vi "Example Feedbacknode 1.vi"() -> ()   [LabVIEW 2014]
panel:
  out "Error Out":errorcluster
  in  "Error In":errorcluster
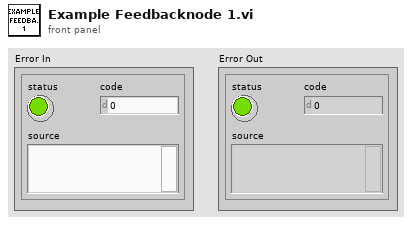
[diagram p1: front panel]
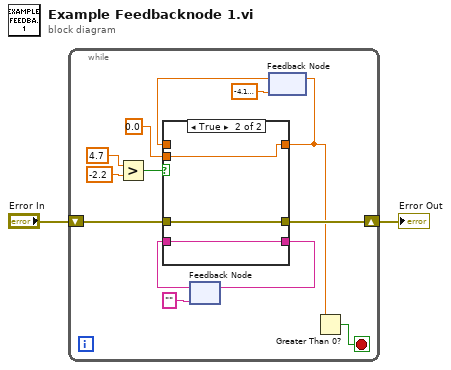
[diagram p0: block diagram]
diagram:
  n1 = while {
    shift-right: [w15] -> w2
    shift-left: "Error In" -> [w14]
    stop <- w4 stop-if-true
    n2 = Greater?(x=4.7, y=-2.2) -> (0:w13:bool)
    n3 = feedback #1("") -> (w6:string)
    n4 = feedback #2(sgl -4.2) -> (w8:sgl)
    n5 = case shown="True" w13 {
      tunnel: [w17 w21] -> w15
      tunnel: w14 -> [w17 w21]
      tunnel: sgl 0.0 -> [_ w20]
      tunnel: [w18 w20] -> w3
      tunnel: w8 -> [w18 _]
      tunnel: [w16 w19] -> w7
      tunnel: w6 -> [w16 w19]
      frame False {
      }
      frame True {
      }
    }
    n6 = feedback-in #1(w7) -> ()
    n7 = feedback-in #2(w3) -> ()
    n8 = Greater Than 0?(x=w3) -> (x > 0?=w4:bool)
  }
  "Error Out" <- w2
